vi "CUST Read Header Data.vi"(10 "pseudoPdcId":i32, 11 "timeoutMs":i32) -> (3 "function return":i32)   [LabVIEW 2017, in "S3DK.lvlib" / "C37118-DLL.lvlib"]
doc: "STRONGRIDIEEEC37118DLL_API int __cdecl readHeaderData( int32_t timeoutMs, int32_t pseudoPdcId);"
uses:
  <vilib>/S3DK/c37118-dll/C37118-DLL.lvlib
  <vilib>/S3DK/data/StrongridDLL.dll
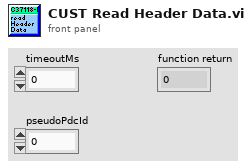
[diagram p1: front panel]
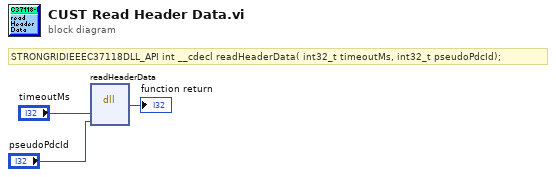
[diagram p0: block diagram]
diagram:
  # "STRONGRIDIEEEC37118DLL_API int __cdecl readHeaderData( int32_t timeoutMs, int32_t pseudoPdcId);"
  n1 = dll-call lib="C:/Program Files/National Instruments/LabVIEW 2017/vi.lib/S3DK/data/StrongridDLL.*" fn="readHeaderData"("timeoutMs"="timeoutMs", "pseudoPdcId"="pseudoPdcId") -> (→"function return":i32)  [unwired: 5 in, 2 out]
